vi "_script_update_JKISM_doc.vi"() -> ()   [LabVIEW 2014]
uses:
  JKI State Machine++.lvlib
panel:
  out "Array":cluster{refnum<vi>, "Text":string}[](array[cluster])
  in  "vi path":path
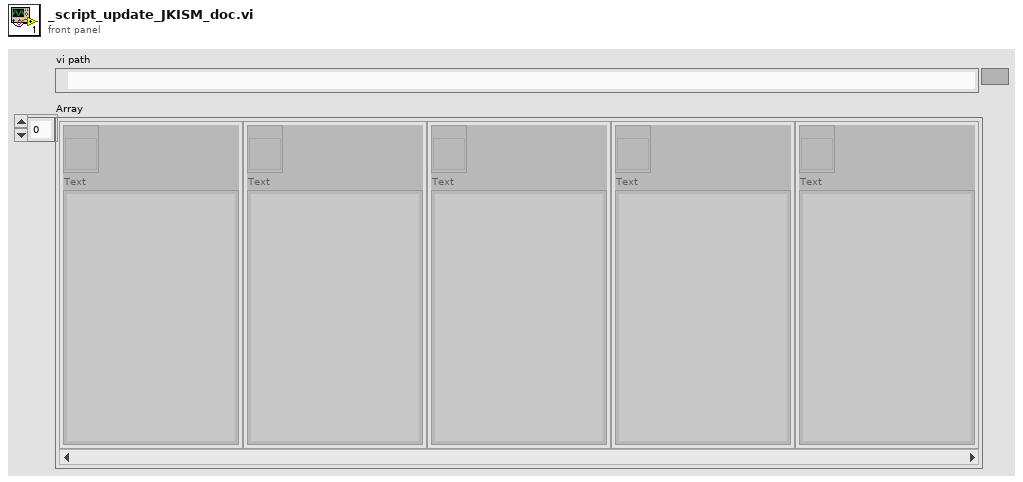
[diagram p1: front panel]
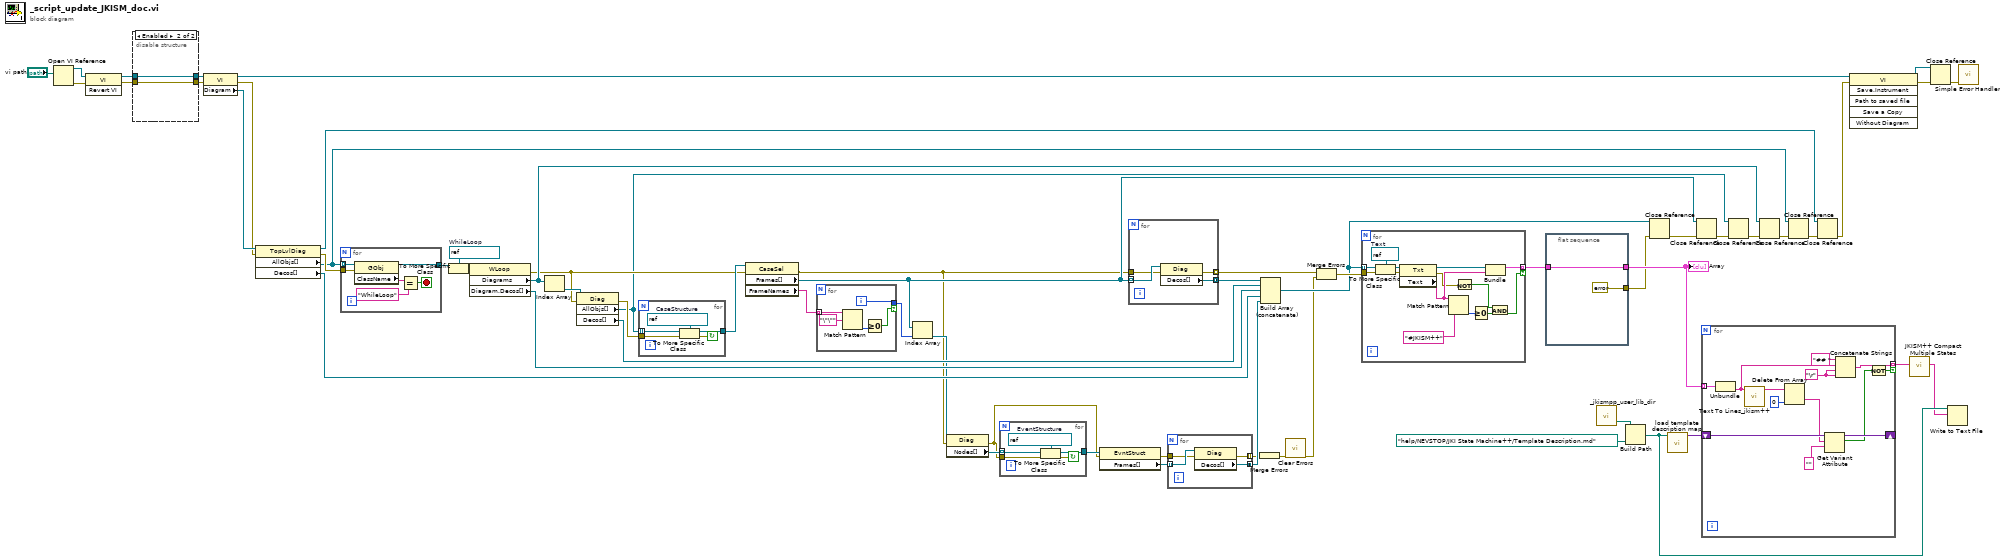
[diagram p0: block diagram]
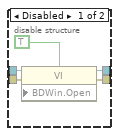
[diagram p2: hidden frame]
diagram:
  w52 = refnum<vi> refnum  # WhileLoop
  n1 = Open VI Reference(vi path="vi path") -> (vi reference=w61:refnum<vi>, error out=w62:errorcluster)  [unwired: 5 in]
  n2 = invoke class="VI" method="Revert VI"(reference=w61, error in=w62) -> (reference out=w44:refnum<vi>, error out=w43:errorcluster)  [unwired: 1 in, 1 out]
  n3 = disable-structure shown="Enabled" {
    disable-tunnel: w44 -> [w67 w69]
    disable-tunnel: w43 -> [w66 w68]
    disable-tunnel: [w65 w69] -> w42
    disable-tunnel: [w64 w68] -> w41
    frame Disabled {
      n4 = property class="VI"(reference=w67, error in=w66, "BDWin.Open"=TRUE ("Block Diagram Window:Open")) -> (reference out=w65:refnum<vi>, error out=w64:errorcluster)
    }
    frame Enabled {
    }
  }
  n5 = property class="VI"(reference=w42, error in=w41) -> (reference out=w60:refnum<vi>, error out=w55:errorcluster, "Diagram"=w56:refnum<vi>)
  n6 = property class="TopLvlDiag"(reference=w56, error in=w55) -> (reference out=w46:refnum<vi>, error out=w54:errorcluster, "AllObjs[]"=w48:refnum<vi>[], "Decos[]"=w15:refnum<vi>[])
  n7 = for {
    tunnel: w48 -> [w75] mode=indexing
    tunnel: w54 -> [w74]
    tunnel: [w73] -> w53
    stop <- w70 stop-if-true
    n8 = property class="GObj"(reference=w75, error in=w74) -> (reference out=w73:refnum<vi>, "ClassName"=w72:string)  [unwired: 1 out]
    n9 = Equal?(x=w72, y="WhileLoop") -> (x = y?=w70:bool)
  }
  n10 = To More Specific Class(target class=w52, reference=w53) -> (specific class reference=w51:refnum<vi>, error out=w50:errorcluster)  [unwired: 1 in]
  n11 = property class="WLoop"(reference=w51, error in=w50) -> (error out=w36:errorcluster, "Diagrams"=w40:refnum<vi>[], "Diagram.Decos[]"=w16:refnum<vi>[])  [unwired: 1 out]
  n12 = Index Array(array=w40) -> (element=w39:refnum<vi>)  [unwired: 1 in]
  n13 = property class="Diag"(reference=w39, error in=w36) -> (error out=w38:errorcluster, "AllObjs[]"=w32:refnum<vi>[], "Decos[]"=w18:refnum<vi>[])  [unwired: 1 out]
  n14 = for {
    tunnel: w32 -> [w80] mode=indexing
    tunnel: w38 -> [w79]
    tunnel: [w77] -> w37
    stop <- w78 continue-if-true
    w76 = refnum<vi> refnum  # CaseStructure
    n15 = To More Specific Class(target class=w76, reference=w80, error in=w79) -> (specific class reference=w77:refnum<vi>, error out=w78:errorcluster)
  }
  n16 = property class="CaseSel"(reference=w37, error in=w36) -> (error out=w4:errorcluster, "Frames[]"=w13:refnum<vi>[], "FrameNames"=w14:string[])  [unwired: 1 out]
  n17 = for {
    tunnel: w14 -> [w85] mode=indexing
    tunnel: [w83] -> w12 if=w81
    i -> [w83]
    n18 = Match Pattern(string=w85, regular expression="\"\"") -> (offset past match=w82:i32)  [unwired: 1 in, 3 out]
    n19 = Greater Or Equal To 0?(x=w82) -> (x >= 0?=w81:bool)
  }
  n20 = Index Array(array=w13, index=w12) -> (element=w11:refnum<vi>)
  n21 = property class="Diag"(reference=w11, error in=w4) -> (error out=w7:errorcluster, "Nodes[]"=w10:refnum<vi>[])  [unwired: 1 out]
  n22 = for {
    tunnel: w10 -> [w90] mode=indexing
    tunnel: w7 -> [w89]
    tunnel: [w87] -> w9
    stop <- w88 continue-if-true
    w86 = refnum<vi> refnum  # EventStructure
    n23 = To More Specific Class(target class=w86, reference=w90, error in=w89) -> (specific class reference=w87:refnum<vi>, error out=w88:errorcluster)
  }
  n24 = property class="EvntStruct"(reference=w9, error in=w7) -> (error out=w6:errorcluster, "Frames[]"=w8:refnum<vi>[])  [unwired: 1 out]
  n25 = for {
    tunnel: w13 -> [w94] mode=indexing
    tunnel: w4 -> [w93]
    tunnel: [w92] -> w23 mode=indexing
    tunnel: [w91] -> w19 mode=concatenating
    n26 = property class="Diag"(reference=w94, error in=w93) -> (error out=w92:errorcluster, "Decos[]"=w91:refnum<vi>[])  [unwired: 1 out]
  }
  n27 = for {
    tunnel: w8 -> [w98] mode=indexing
    tunnel: w6 -> [w97]
    tunnel: [w96] -> w3 mode=indexing
    tunnel: [w95] -> w5 mode=concatenating
    n28 = property class="Diag"(reference=w98, error in=w97) -> (error out=w96:errorcluster, "Decos[]"=w95:refnum<vi>[])  [unwired: 1 out]
  }
  n29 = Merge Errors(w3) -> (w2:errorcluster)
  n30 = Build Array (concatenate)(w19, w18, w16, w15, w5) -> (w17:refnum<vi>[])
  n31 = call <vilib>:"Clear Errors.vi"("error in (no error)"=w2) -> ("error out"=w1:errorcluster)  [unwired: 5 in, 1 out]
  n32 = Merge Errors(w23, w1) -> (w20:errorcluster)
  n33 = for {
    tunnel: w17 -> [w112] mode=indexing
    tunnel: w20 -> [w111]
    tunnel: [w105] -> w22 mode=indexing if=w101
    w110 = refnum<vi> refnum  # Text
    n34 = To More Specific Class(target class=w110, reference=w112, error in=w111) -> (specific class reference=w109:refnum<vi>, error out=w107:errorcluster)
    n35 = property class="Txt"(reference=w109, error in=w107) -> (reference out=w108:refnum<vi>, error out=w100:errorcluster, "Text"=w104:string)
    n36 = Match Pattern(string=w104, regular expression="#JKISM++") -> (offset past match=w103:i32)  [unwired: 1 in, 3 out]
    n37 = Not(x=w100) -> (.not. x?=w99:bool)
    n38 = Greater Or Equal To 0?(x=w103) -> (x >= 0?=w102:bool)
    n39 = Bundle(w108, "Text"=w104) -> (w105:cluster{refnum<vi>, "Text":string})  [unwired: 1 in]
    n40 = And(x=w99, y=w102) -> (x .and. y?=w101:bool)
  }
  n41 = flat-sequence {
    tunnel: w22 -> [w113]
    tunnel: [errorcluster {"status"=FALSE, "code"=0, "source"=""} ("error in (no error)")] -> w21
    tunnel: [w113] -> w27
    frame #0 {
    }
  }
  n42 = call "_jkismpp_user_lib_dir.vi"() -> ("<LabVIEW>"=w29:path)  [unwired: 2 in, 1 out]
  n43 = Build Path(base path=w29, name or relative path=path "help/NEVSTOP/JKI State Machine++/Template Description.md" ("Path")) -> (appended path=w25:path)
  n44 = Close Reference(reference=w17, error in (no error)=w21) -> (error out=w35:errorcluster)
  n45 = call "load template description map.vi"("Path"=w25) -> ("variant"=w28:variant)  [unwired: 9 in, 1 out]
  n46 = Close Reference(reference=w13, error in (no error)=w35) -> (error out=w34:errorcluster)
  n47 = for {
    shift-right: [w126] -> _
    shift-left: w28 -> [w127]
    tunnel: w27 -> [w125] mode=indexing
    tunnel: [w117] -> w26 mode=indexing if=w118
    w116 = "\r"
    n48 = Unbundle(w125) -> ("Text"=w120:string)  [unwired: 1 out]
    n49 = call "Text To Lines_jkism++.vi"("string"=w120) -> ("Lines"=w124:string[])  [unwired: 9 in, 1 out]
    n50 = Delete From Array(array=w124, index=0) -> (deleted portion=w122:string)  [unwired: 1 in, 1 out]
    n51 = Get Variant Attribute(Variant=w127, name=w122, default value (empty Variant)="" ("deleted portion")) -> (duplicate Variant=w126:variant, found=w119:bool)  [unwired: 1 in, 2 out]
    n52 = Concatenate Strings("## " ("string"), w120, w116, w116) -> (w117:string)
    n53 = Not(x=w119) -> (.not. x?=w118:bool)
  }
  n54 = Close Reference(reference=w32, error in (no error)=w34) -> (error out=w33:errorcluster)
  n55 = Close Reference(reference=w40, error in (no error)=w33) -> (error out=w49:errorcluster)
  n56 = Close Reference(reference=w48, error in (no error)=w49) -> (error out=w47:errorcluster)
  n57 = Close Reference(reference=w46, error in (no error)=w47) -> (error out=w45:errorcluster)
  n58 = invoke class="VI" method="Save.Instrument"(reference=w60, error in=w45) -> (reference out=w58:refnum<vi>, error out=w59:errorcluster)  [unwired: 4 in, 4 out]
  n59 = call "JKISM++ Compact Multiple States.vi"("States in Lines"=w26) -> ("States"=w24:string)  [unwired: 9 in]
  n60 = Close Reference(reference=w58, error in (no error)=w59) -> (error out=w57:errorcluster)
  n61 = Write to Text File(file (use dialog)=w25, text=w24) -> ()  [unwired: 2 in, 3 out]
  n62 = call <vilib>:"Simple Error Handler.vi"("error in (no error)"=w57) -> ()  [unwired: 4 in, 5 out]
  "Array" <- w27
